vi "generate_stimulus_array.vi"(1 "Values Cluster":T1) -> (0 "Array":dbl[](array[numeric]))   [LabVIEW 2015]
uses:
  <vilib>/gmath/statdist.llb/Exp Random.vi
  <vilib>/gmath/NI_Gmath.lvlib
panel:
  in  "Minimum time between stimuli (ms)":i32=2000
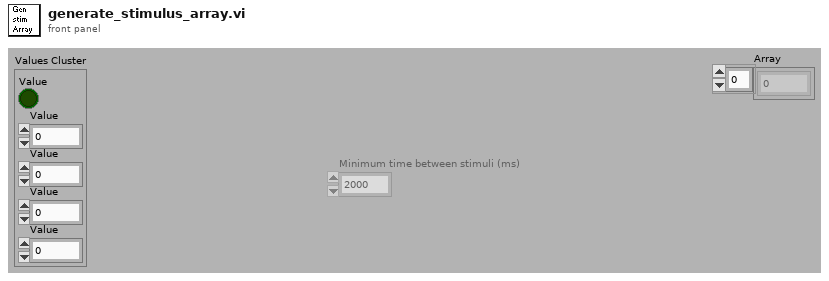
[diagram p1: front panel]
types:
  T1 = cluster{"Value":bool, "Value":dbl, "Value":dbl, "Value":dbl, "Value":u16}
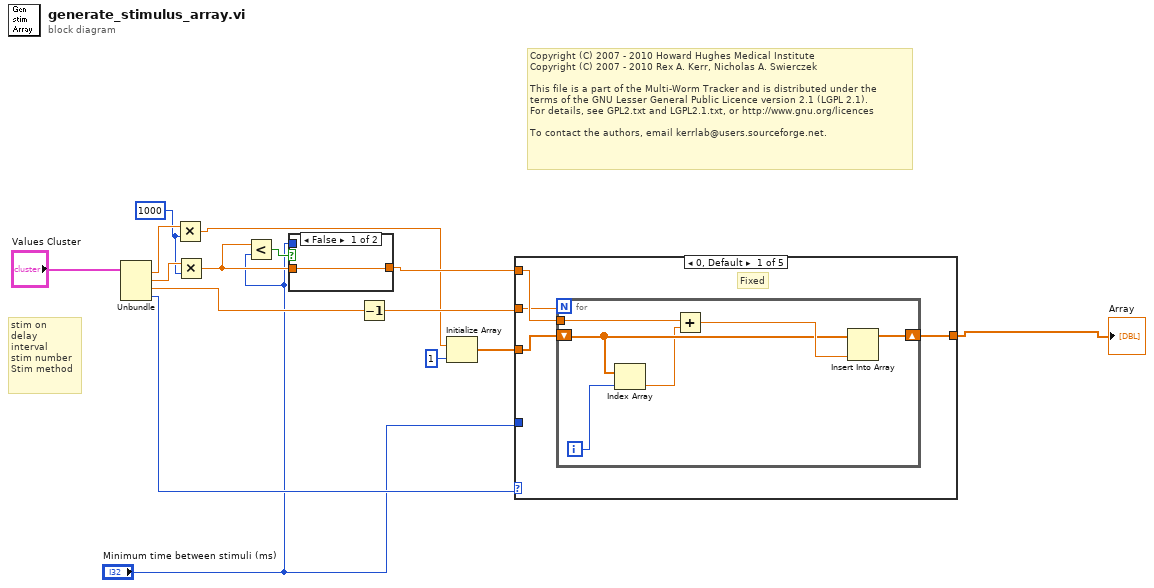
[diagram p0: block diagram]
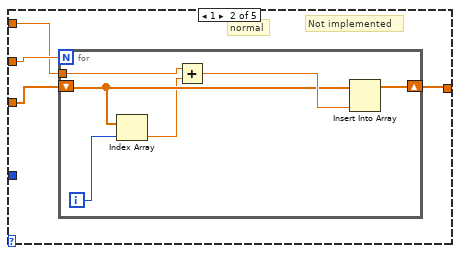
[diagram p3: hidden frame]
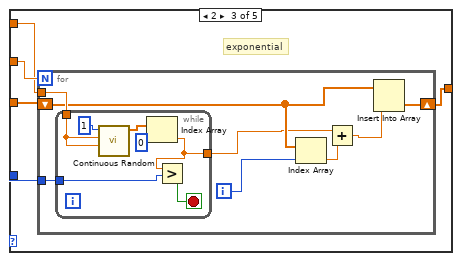
[diagram p4: hidden frame]
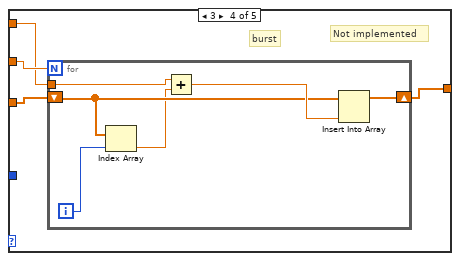
[diagram p5: hidden frame]
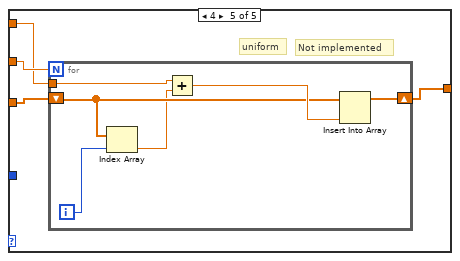
[diagram p6: hidden frame]
diagram:
  w9 = 1000
  # "stim on\ndelay\ninterval\nstim number\nStim method"
  # "Copyright (C) 2007 - 2010 Howard Hughes Medical Institute\nCopyright (C) 2007 - 2010 Rex A. Kerr, Nicholas A. Swierczek\n \nThis file is a part of the Multi-Worm Tracker and is distributed under the\nterms of the GNU Lesser General Public Licence version 2.1 (LGPL 2.1).\nFor details, see GPL2.txt and LGPL2.1.txt, or http://www.gnu.org/licences\n \nTo contact the authors, email kerrlab@users.sourceforge.net."
  n1 = Unbundle("Values Cluster") -> ("Value"=w11:dbl, "Value"=w10:dbl, "Value"=w13:dbl, "Value"=w12:u16)  [unwired: 1 out]
  n2 = Multiply(x=w11, y=w9) -> (x*y=w5:dbl)
  n3 = Multiply(x=w10, y=w9) -> (x*y=w2:dbl)
  n4 = Less?(x=w2, y="Minimum time between stimuli (ms)") -> (x < y?=w8:bool)
  n5 = case shown="False" w8 {
    tunnel: w2 -> [w16 _]
    tunnel: [w16 w17] -> w7
    tunnel: "Minimum time between stimuli (ms)" -> [_ w17]
    frame False {
    }
    frame True {
    }
  }
  n6 = Decrement(x=w13) -> (x-1=w15:dbl)
  n7 = Initialize Array(w5, 1 ("dimension size")) -> (w4:dbl[])
  n8 = case shown="0, Default" w12 {
    tunnel: w7 -> [w21 w29 w40 w58 w68]
    tunnel: w15 -> [w20 w30 w42 w59 w69]
    tunnel: [w19 w28 w41 w61 w71] -> w3
    tunnel: "Minimum time between stimuli (ms)" -> [_ _ w39 _ _]
    tunnel: w4 -> [w18 w31 w38 w60 w70]
    frame 0, Default {
      # "Fixed"
      n9 = for {
        N: w20 -> [_]
        tunnel: w21 -> [w27]
        shift-right: [w26] -> w19
        shift-left: w18 -> [w24]
        i -> [w23]
        n10 = Index Array(array=w24, index=w23) -> (element=w22:dbl)
        n11 = Add(x=w27, y=w22) -> (x+y=w25:dbl)
        n12 = Insert Into Array(array=w24, new element=w25) -> (w26:dbl[])  [unwired: 1 in]
      }
    }
    frame 1 {
      # "Not implemented"
      # "normal"
      n13 = for {
        N: w30 -> [_]
        shift-right: [w37] -> w28
        shift-left: w31 -> [w35]
        tunnel: w29 -> [w32]
        i -> [w34]
        n14 = Index Array(array=w35, index=w34) -> (element=w33:dbl)
        n15 = Add(x=w32, y=w33) -> (x+y=w36:dbl)
        n16 = Insert Into Array(array=w35, new element=w36) -> (w37:dbl[])  [unwired: 1 in]
      }
    }
    frame 2 {
      # "exponential"
      n17 = for {
        N: w42 -> [_]
        tunnel: w40 -> [w49]
        shift-right: [w50] -> w41
        shift-left: w38 -> [w48]
        tunnel: w39 -> [w46]
        i -> [w43]
        n18 = while {
          tunnel: w49 -> [w56]
          tunnel: w46 -> [w52]
          tunnel: [w51] -> w45
          stop <- w53 stop-if-true
          n19 = call-poly <vilib>:"Continuous Random.vi"("b"=w56, "a"=w56, "samples"=1) -> ("exp random data"=w55:dbl[])  [unwired: 7 in, 1 out]
          n20 = Index Array(array=w55, index=0) -> (element=w51:dbl)
          n21 = Greater?(x=w51, y=w52) -> (0:w53:bool)
        }
        n22 = Index Array(array=w48, index=w43) -> (element=w44:dbl)
        n23 = Add(x=w45, y=w44) -> (x+y=w47:dbl)
        n24 = Insert Into Array(array=w48, new element=w47) -> (w50:dbl[])  [unwired: 1 in]
      }
    }
    frame 3 {
      # "Not implemented"
      # "burst"
      n25 = for {
        N: w59 -> [_]
        shift-right: [w67] -> w61
        shift-left: w60 -> [w65]
        tunnel: w58 -> [w62]
        i -> [w64]
        n26 = Index Array(array=w65, index=w64) -> (element=w63:dbl)
        n27 = Add(x=w62, y=w63) -> (x+y=w66:dbl)
        n28 = Insert Into Array(array=w65, new element=w66) -> (w67:dbl[])  [unwired: 1 in]
      }
    }
    frame 4 {
      # "Not implemented"
      # "uniform"
      n29 = for {
        N: w69 -> [_]
        shift-right: [w77] -> w71
        shift-left: w70 -> [w75]
        tunnel: w68 -> [w72]
        i -> [w74]
        n30 = Index Array(array=w75, index=w74) -> (element=w73:dbl)
        n31 = Add(x=w72, y=w73) -> (x+y=w76:dbl)
        n32 = Insert Into Array(array=w75, new element=w76) -> (w77:dbl[])  [unwired: 1 in]
      }
    }
  }
  "Array" <- w3
